vi "mask.vi"() -> ()   [LabVIEW 2023]
uses:
  global.vi
panel:
  in  "maska":bool[](array[boolean])
  out "tablica maskowana":bool[](array[boolean])
  out "tablica wejsciowa":bool[](array[boolean])
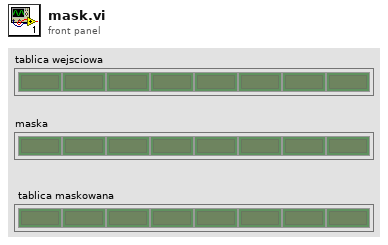
[diagram p1: front panel]
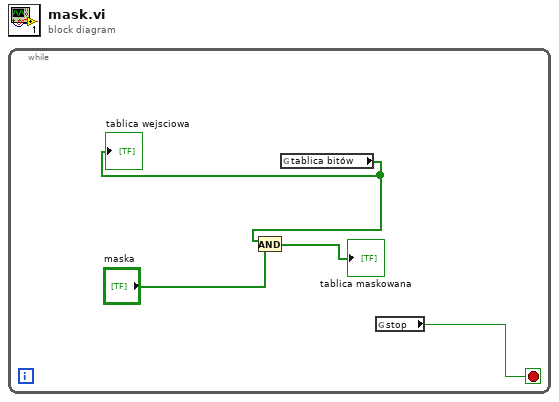
[diagram p0: block diagram]
diagram:
  n1 = while {
    stop <- w1 stop-if-true
    n2 = global read "global.vi" "tablica bitów"() -> (w4:bool[])
    "tablica wejsciowa" <- w4
    n3 = And(x=w4, y="maska") -> (x .and. y?=→"tablica maskowana":bool[])
    n4 = global read "global.vi" "stop"() -> (w1:bool)
  }
